vi "SPCC assignment Client.vi"() -> ()   [LabVIEW 2020]
uses:
  Control03.ctl
  Control01.ctl
  Control02.ctl
  <vilib>/regexp/Match Regular Expression.xnode
panel:
  out "error out 5":errorcluster
  out "error out 4":errorcluster
  out "error out 3":errorcluster
  out "error out 2":errorcluster
  out "Enter":T1=enum."disable"
  out "Account number":string
  out "error out":errorcluster
  out "Right Menu 2":string
  out "ATM":string
  out "Right Menu 3":string
  out "Right Menu 1":string
  out "Left Menu 3":string
  out "Left Menu 2":string
  out "Left Menu 1":string
  in  "Right Button 2":bool
  in  "Right Button 3":bool
  in  "Right Button 1":bool
  in  "Left Button 2":bool
  in  "Left Button 3":bool
  in  "Left Button 1":bool
  in  "Enter":bool
  in  "User Input":string
  in  "Card Simulator":bool
  # "ATM Messages"
  # "Right Menu"
  # "Right Buttons"
  # "Left Buttons"
  # "Left Menu"
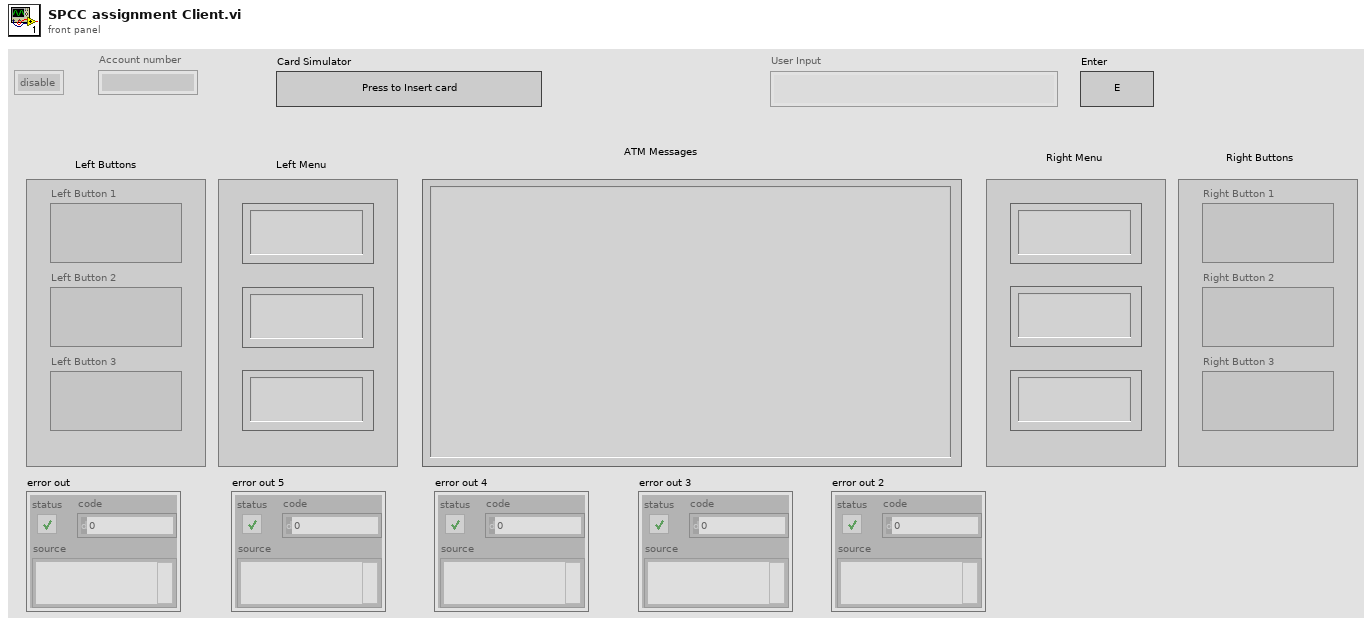
[diagram p1: front panel]
types:
  T1 = typedef "Control03.ctl" = enum16{"withdraw", "deposit", "disable"}
  T2 = typedef "Control01.ctl" = enum16{"Sign in machine", "Start machine", "Welcome "}
  T3 = enum8{"Enabled", "Disabled", "Disabled and Grayed Out"}
  T4 = typedef "Control02.ctl" = enum16{"Start machine", "Welcome "}
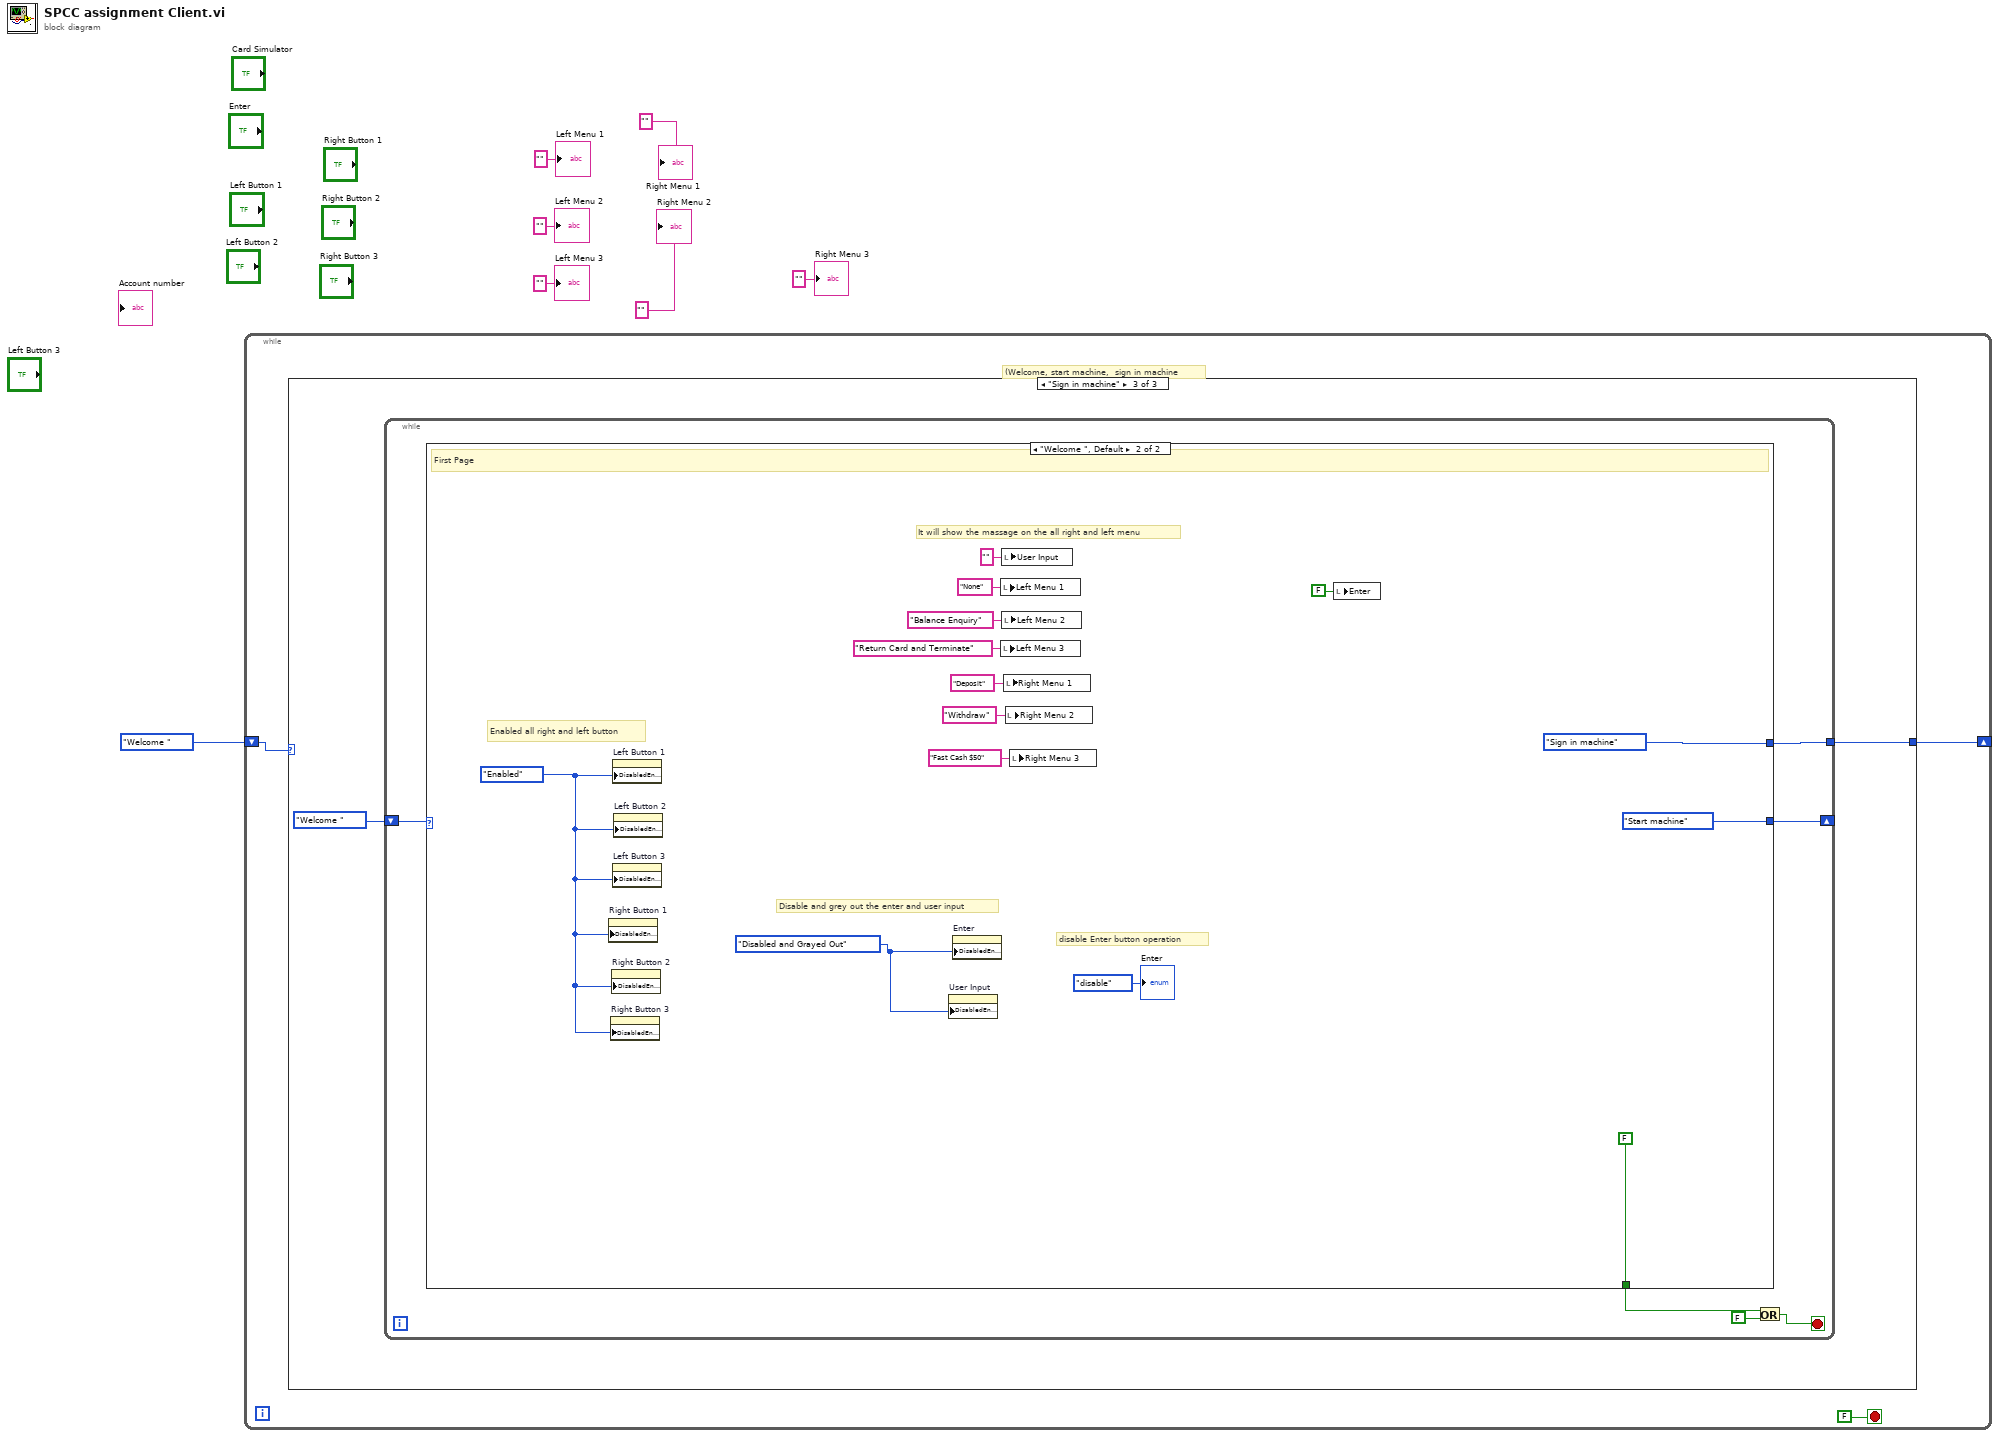
[diagram p0: block diagram]
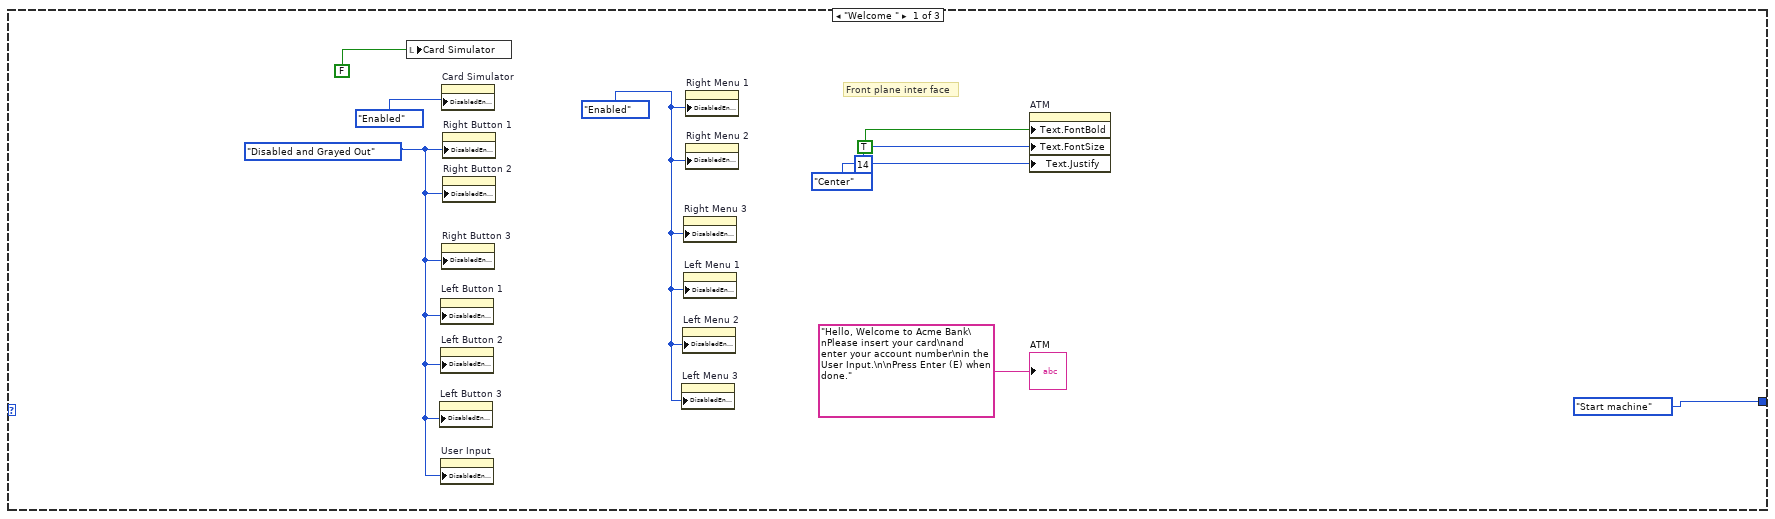
[diagram p2: hidden frame]
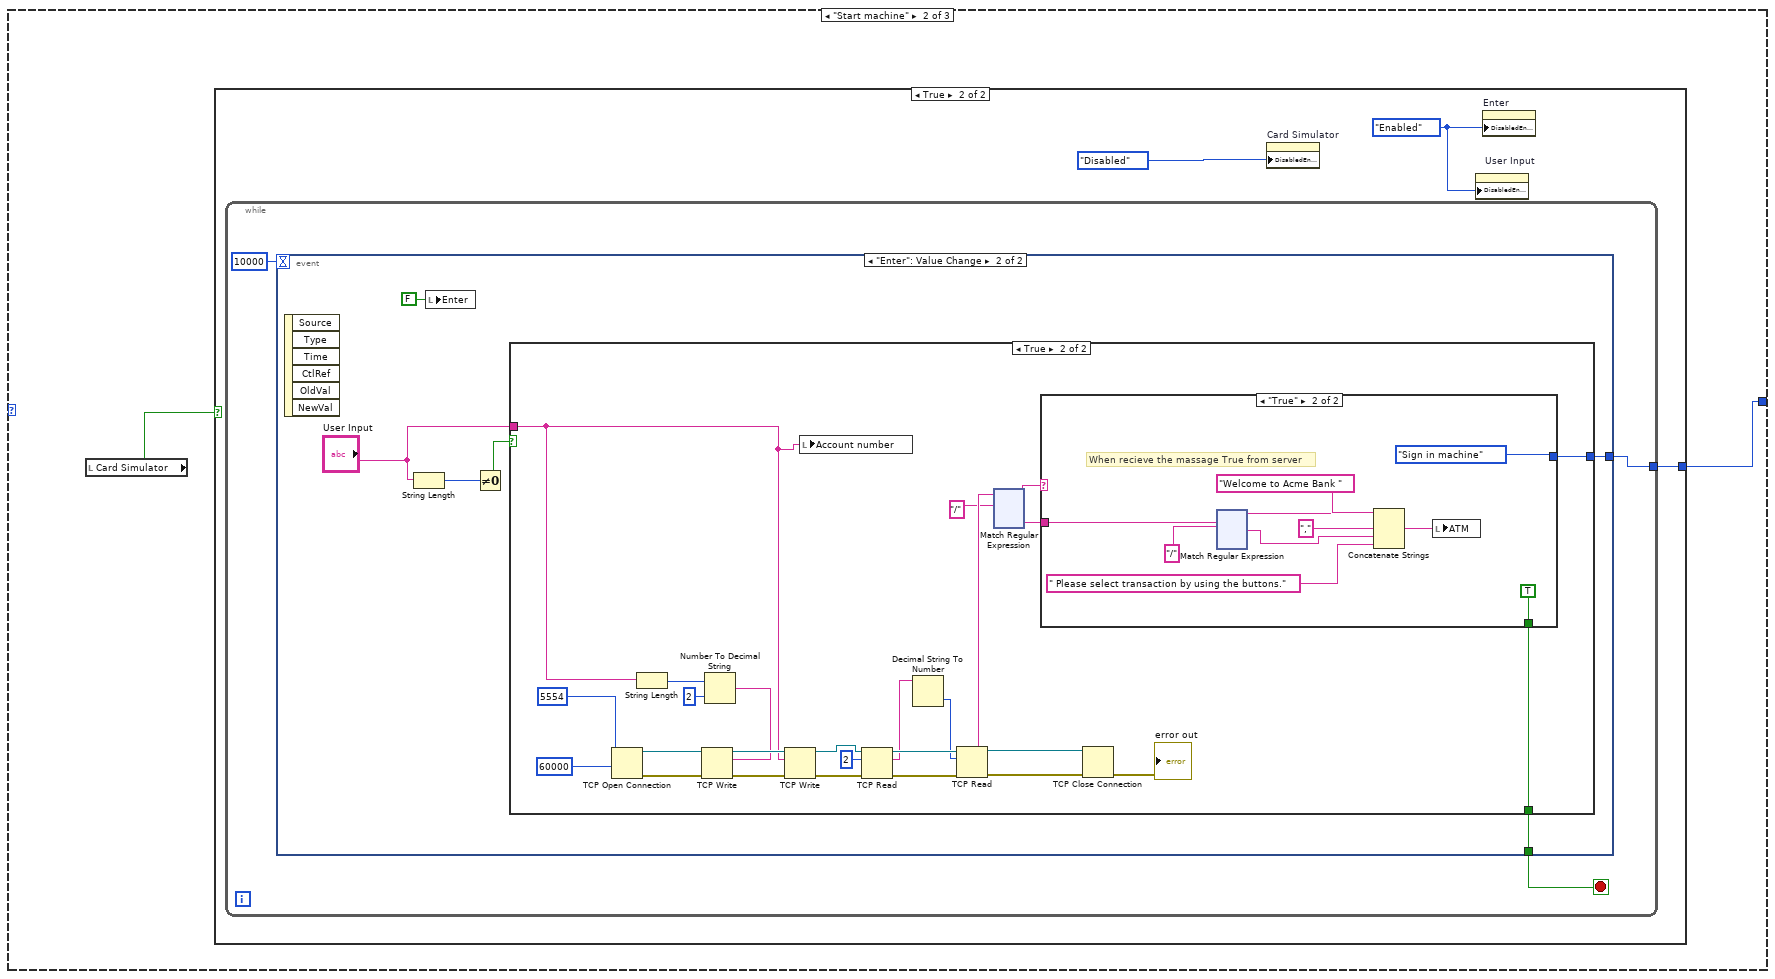
[diagram p3: hidden frame]
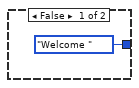
[diagram p4: hidden frame]
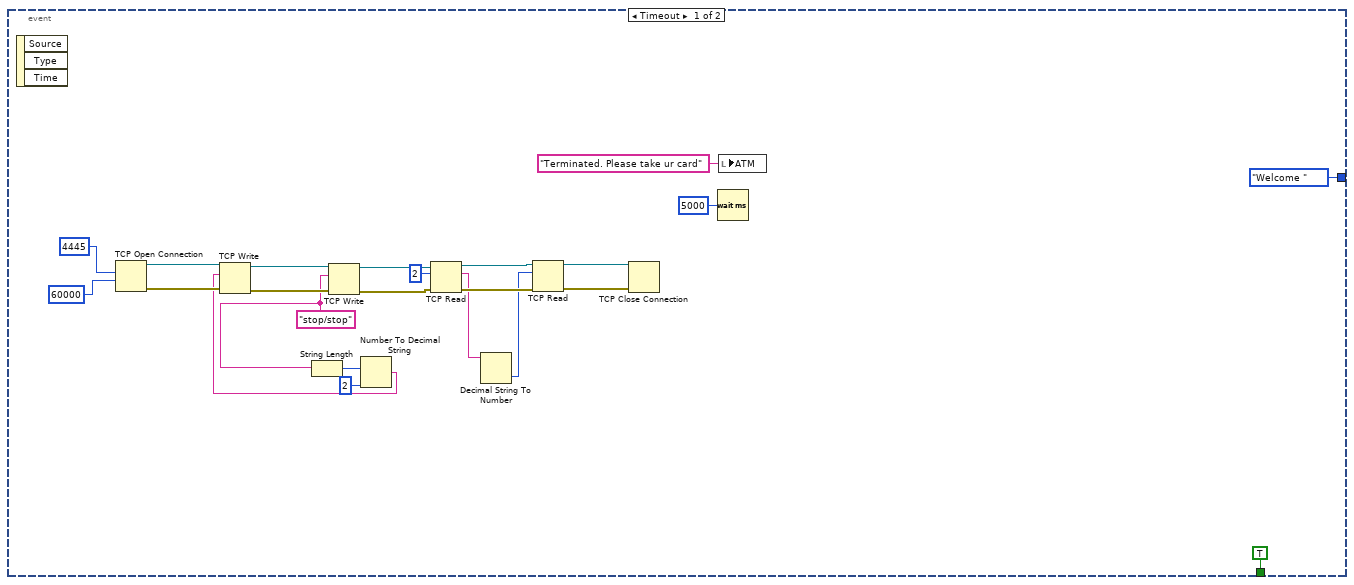
[diagram p5: hidden frame]
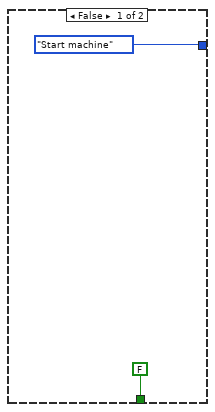
[diagram p6: hidden frame]
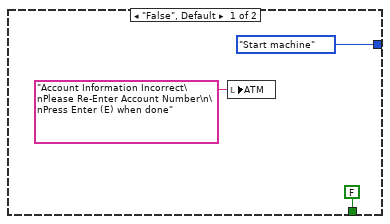
[diagram p7: hidden frame]
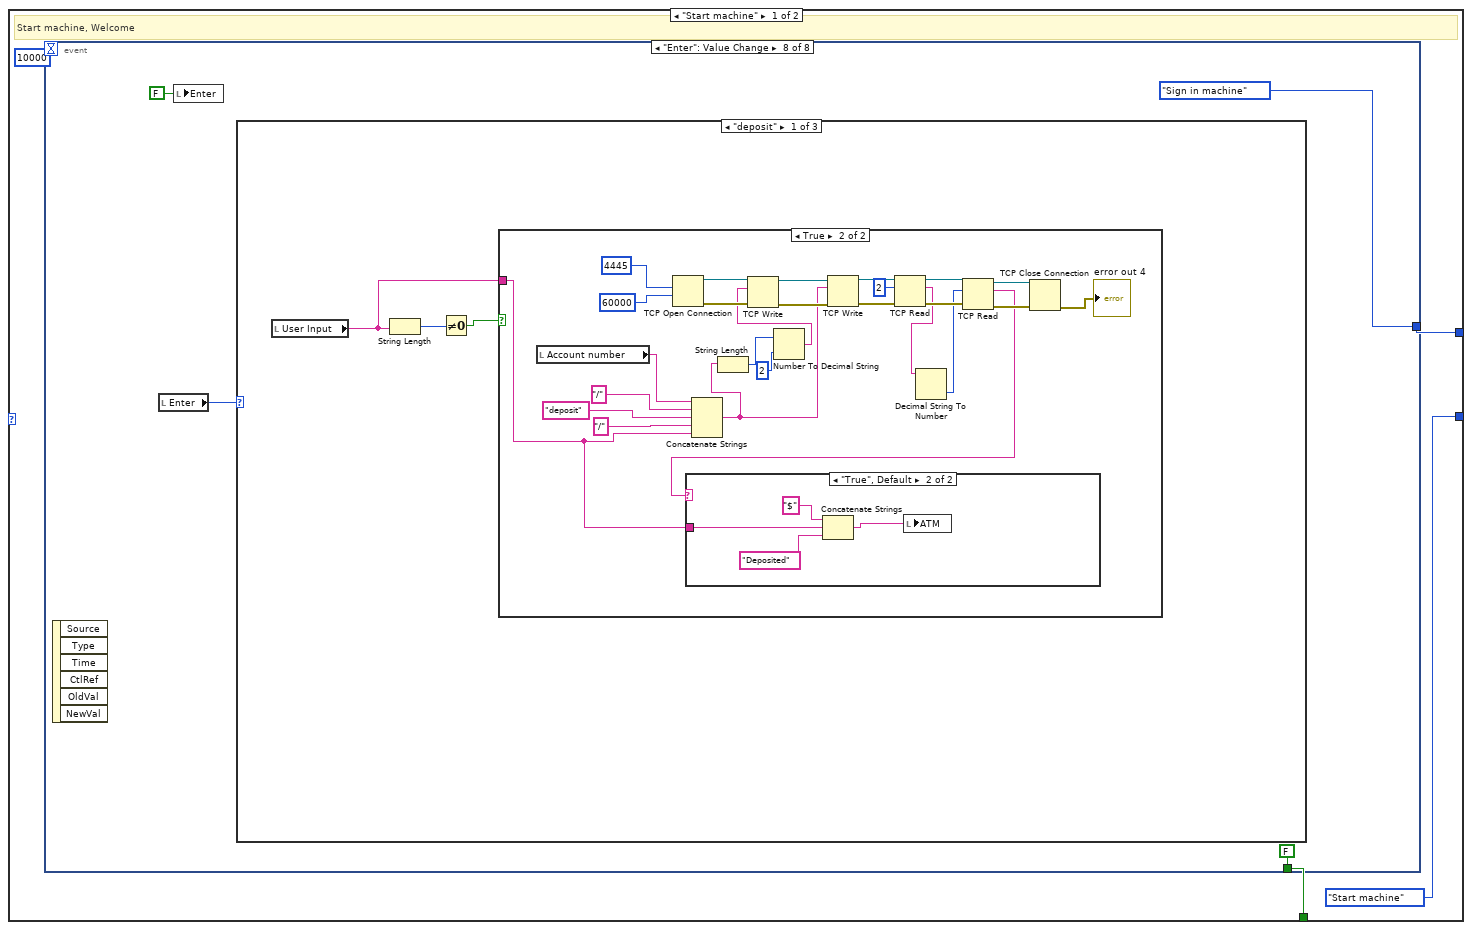
[diagram p8: hidden frame]
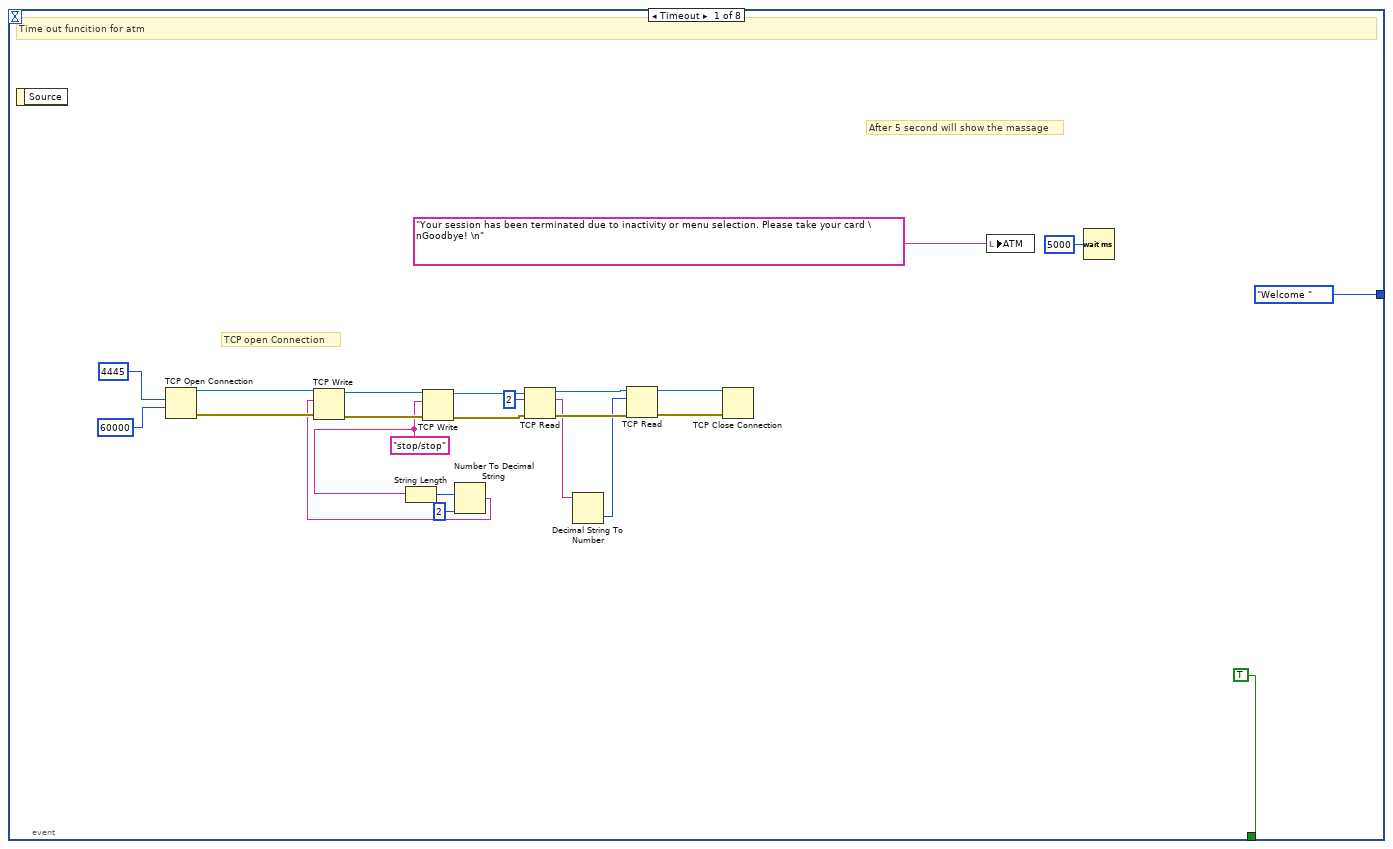
[diagram p9: hidden frame]
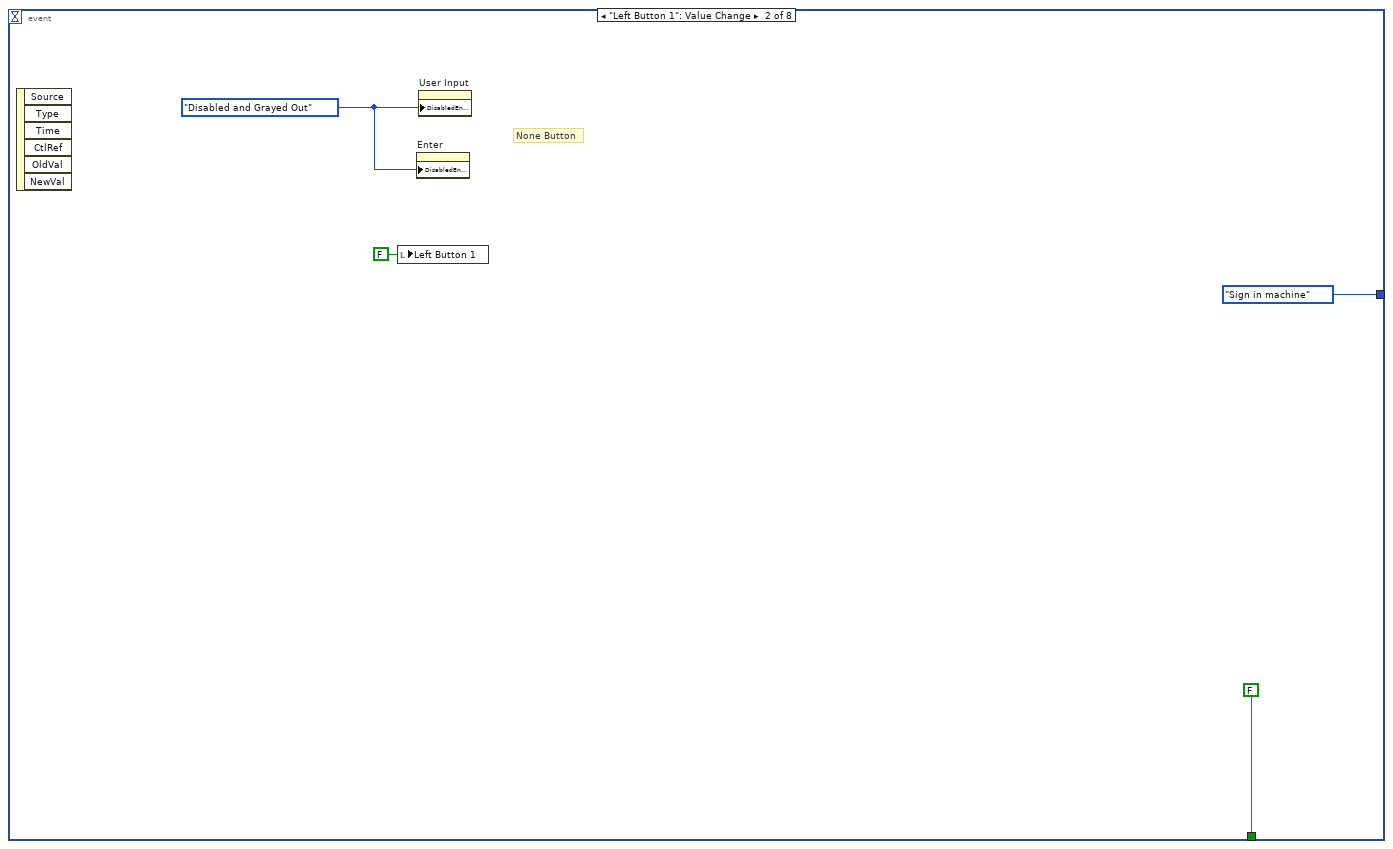
[diagram p10: hidden frame]
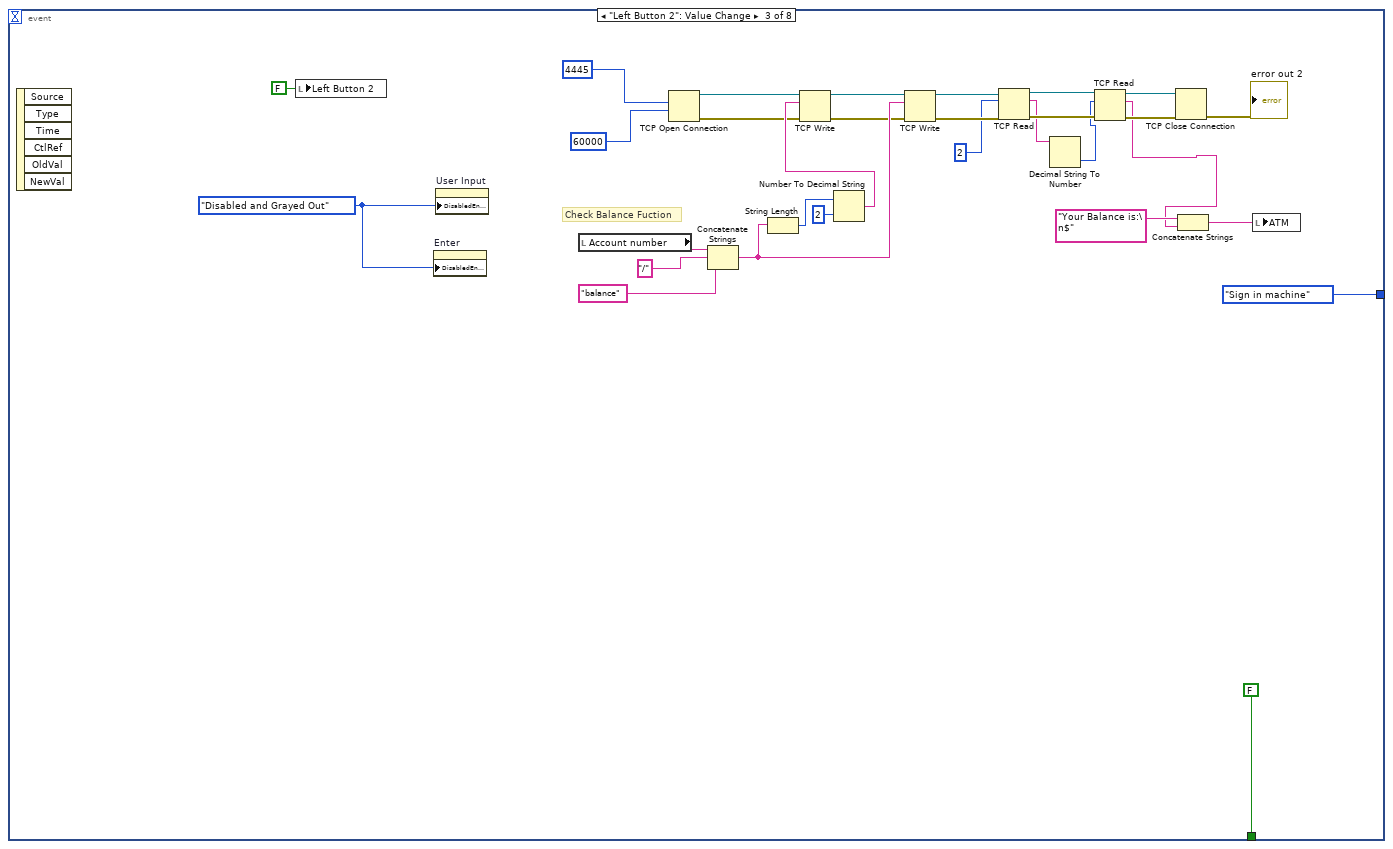
[diagram p11: hidden frame]
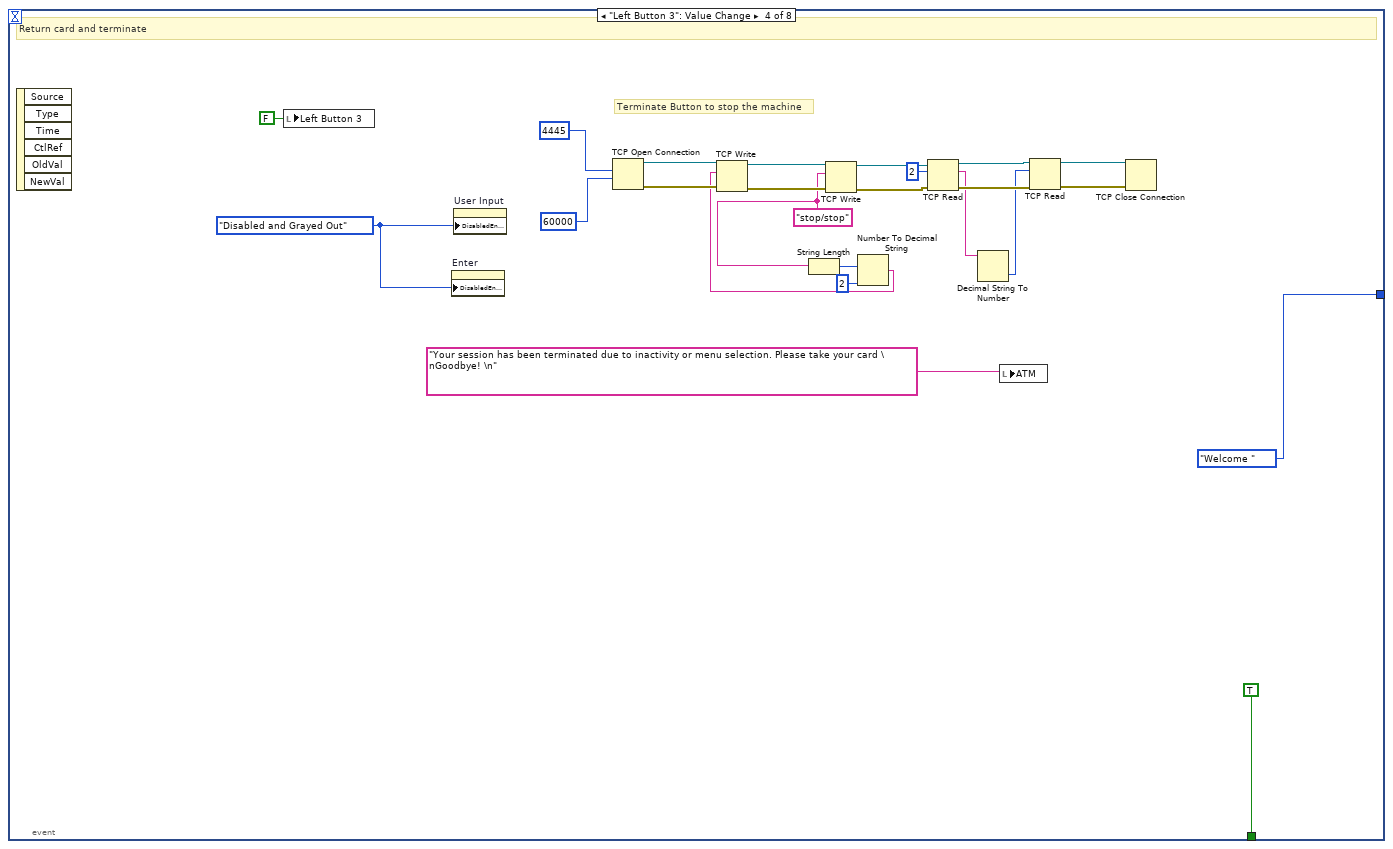
[diagram p12: hidden frame]
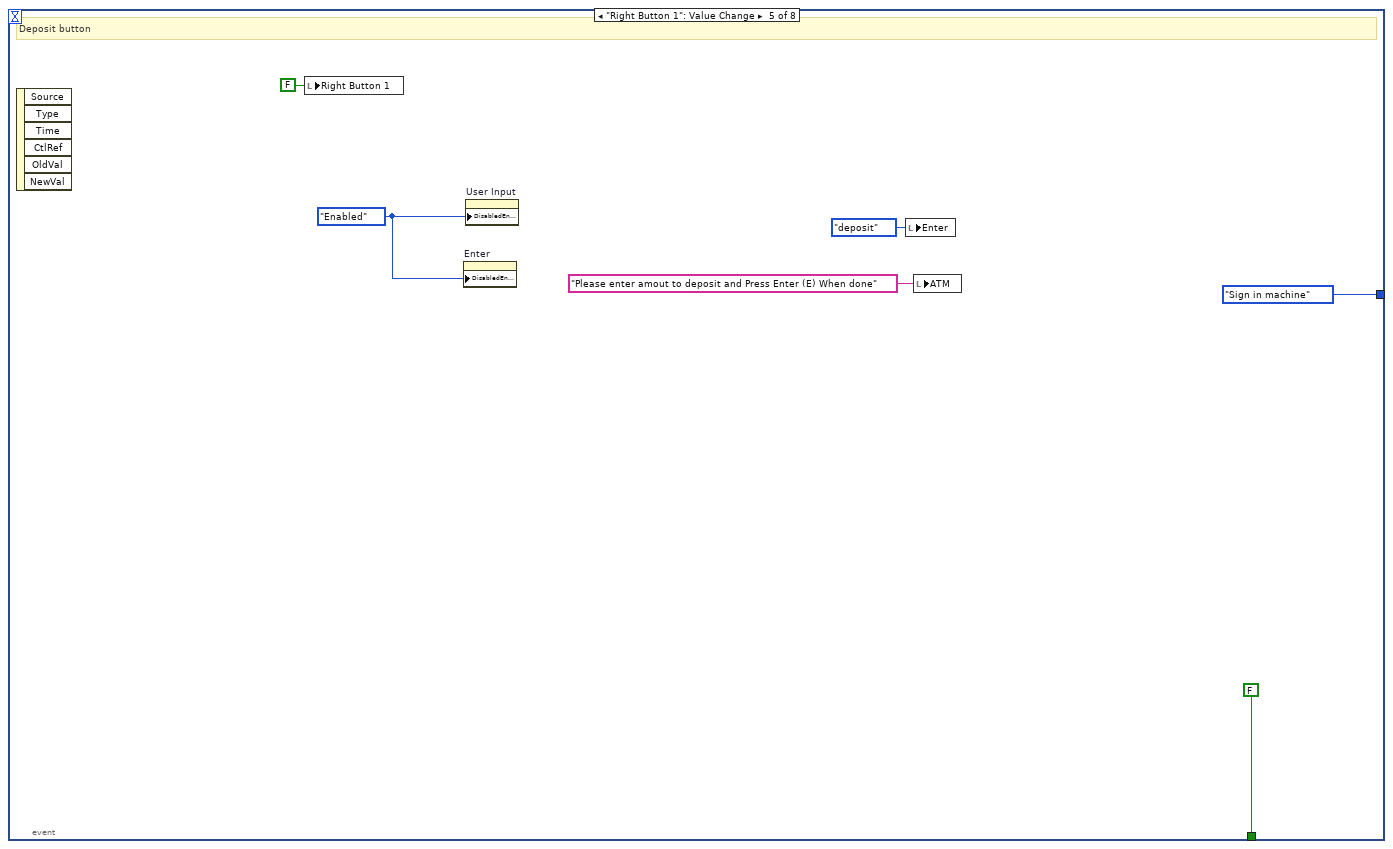
[diagram p13: hidden frame]
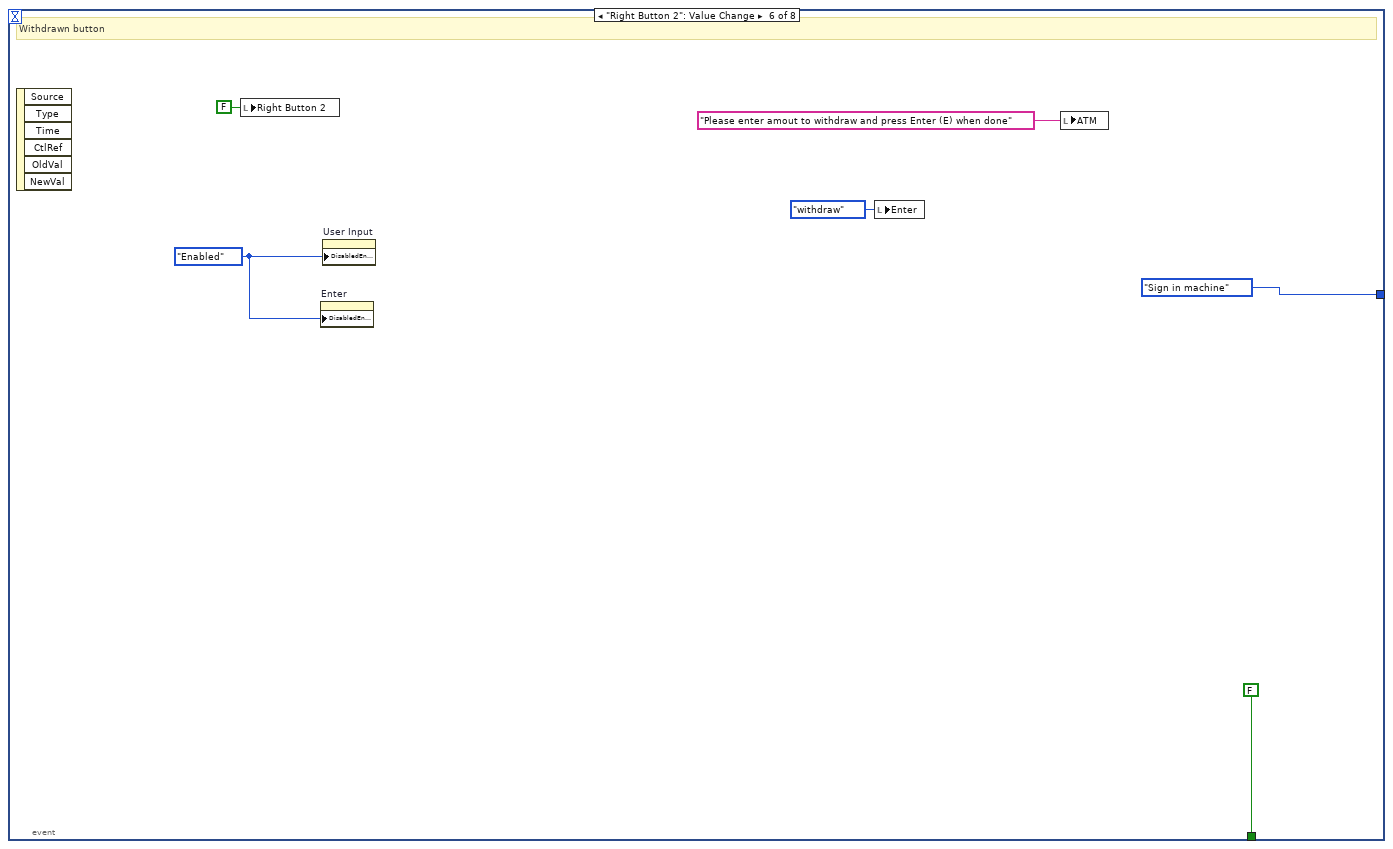
[diagram p14: hidden frame]
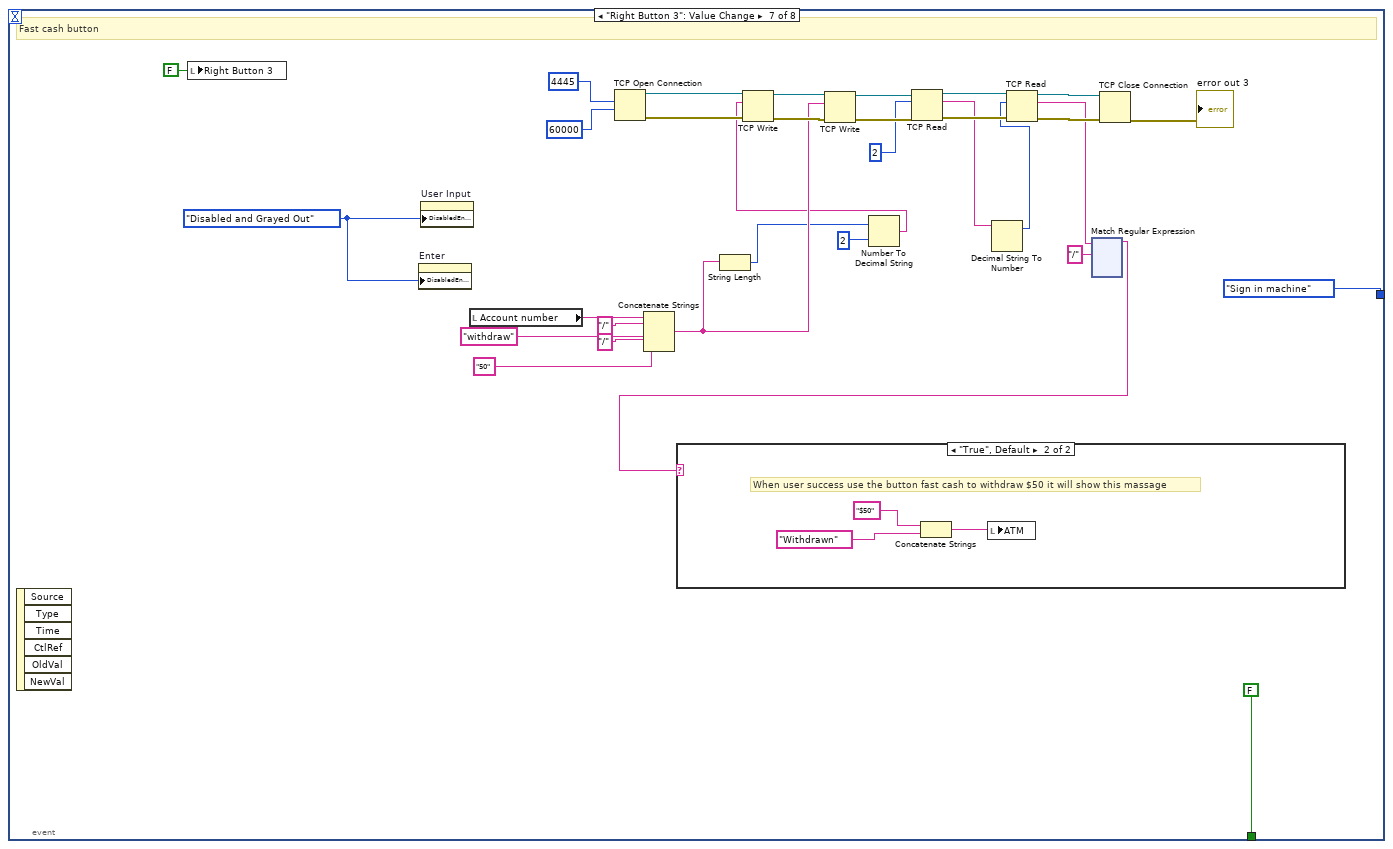
[diagram p15: hidden frame]
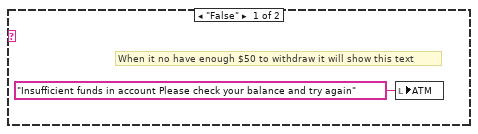
[diagram p16: hidden frame]
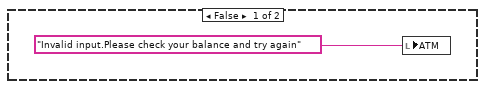
[diagram p17: hidden frame]
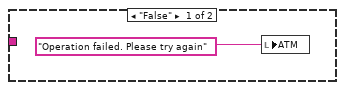
[diagram p18: hidden frame]
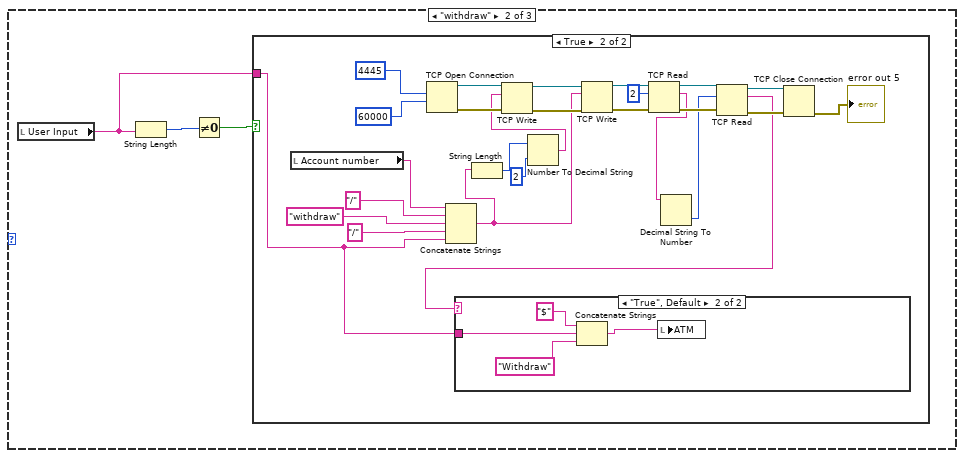
[diagram p19: hidden frame]
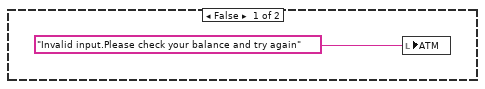
[diagram p20: hidden frame]
diagram:
  n1 = while {
    shift-right: [w8] -> _
    shift-left: Control01."Welcome " ("Enum") -> [w9]
    stop <- FALSE stop-if-true
    # "(Welcome, start machine,  sign in machine"
    n2 = case shown="\"Sign in machine\"" w9 {
      tunnel: [Control01."Start machine" ("Enum") w20 w327] -> w8
      frame "Welcome " {
        w17 = T3."Enabled" ("Disabled")
        w18 = T3."Disabled and Grayed Out" ("Disabled")
        # "Front plane inter face"
        n3 = local write "Card Simulator"(FALSE ("Card Simulator")) -> ()
        n4 = property on="Left Button 3" class="Bool (strict)"("DisabledEnum"=w18) -> ()  [unwired: 2 in, 2 out]
        n5 = property on="Left Button 1" class="Bool (strict)"("DisabledEnum"=w18) -> ()  [unwired: 2 in, 2 out]
        n6 = property on="Left Button 2" class="Bool (strict)"("DisabledEnum"=w18) -> ()  [unwired: 2 in, 2 out]
        n7 = property on="User Input" class="Str"("DisabledEnum"=w18) -> ()  [unwired: 2 in, 2 out]
        n8 = property on="Card Simulator" class="Bool (strict)"("DisabledEnum"=T3."Enabled" ("Disabled")) -> ()  [unwired: 2 in, 2 out]
        n9 = property on="Right Button 3" class="Bool (strict)"("DisabledEnum"=w18) -> ()  [unwired: 2 in, 2 out]
        n10 = property on="Right Button 1" class="Bool (strict)"("DisabledEnum"=w18) -> ()  [unwired: 2 in, 2 out]
        n11 = property on="Right Button 2" class="Bool (strict)"("DisabledEnum"=w18) -> ()  [unwired: 2 in, 2 out]
        n12 = property on="Left Menu 3" class="Str"("DisabledEnum"=w17) -> ()  [unwired: 2 in, 2 out]
        n13 = property on="Left Menu 2" class="Str"("DisabledEnum"=w17) -> ()  [unwired: 2 in, 2 out]
        n14 = property on="Right Menu 3" class="Str"("DisabledEnum"=w17) -> ()  [unwired: 2 in, 2 out]
        n15 = property on="Left Menu 1" class="Str"("DisabledEnum"=w17) -> ()  [unwired: 2 in, 2 out]
        n16 = property on="Right Menu 1" class="Str"("DisabledEnum"=w17) -> ()  [unwired: 2 in, 2 out]
        n17 = property on="Right Menu 2" class="Str"("DisabledEnum"=w17) -> ()  [unwired: 2 in, 2 out]
        n18 = property on="ATM" class="Str"("Text.FontBold"=TRUE ("Text.Font:Bold"), "Text.FontSize"=u32 14 ("Text.Font:Size"), "Text.Justify"=enum16{"Left", "Center", "Right"}."Center" ("Text.Justification")) -> ()  [unwired: 2 in, 2 out]
        "ATM" <- "Hello, Welcome to Acme Bank\nPlease insert your card\nand enter your account number\nin the User Input.\n\nPress Enter (E) when done." ("ATM")
      }
      frame "Start machine" {
        n19 = local read "Card Simulator"() -> (w21:bool)
        n20 = case shown="True" w21 {
          tunnel: [Control01."Welcome " ("Enum") w23] -> w20
          frame False {
          }
          frame True {
            w25 = T3."Enabled" ("Disabled")
            n21 = while {
              tunnel: [w28] -> w23
              stop <- w27 stop-if-true
              n22 = event shown="[1] \"Enter\": Value Change" {
                selector: _ -> [_ _]
                dyn-events: _ -> [_ _]
                timeout: 10000 -> [_ _]
                tunnel: [Control01."Welcome " ("Enum") w54] -> w28
                tunnel: [TRUE w53] -> w27
                event Timeout {
                  w36 = "stop/stop" ("data in")
                  n23 = event-data() -> ()  [unwired: 1 in, 3 out]
                  n24 = TCP Open Connection(remote port or service name=u16 4445, timeout ms (60000)=60000) -> (connection ID=w37:refnum<k5>, error out=w47:errorcluster)  [unwired: 3 in]
                  n25 = String Length(string=w36) -> (length=w31:i32)
                  n26 = Number To Decimal String(number=w31, width (-)=i16 2) -> (decimal integer string=w35:string)
                  n27 = TCP Write(connection ID=w37, data in=w35, error in (no error)=w47) -> (connection ID out=w42:refnum<k5>, error out=w46:errorcluster)  [unwired: 1 in, 1 out]
                  n28 = TCP Write(connection ID=w42, data in=w36, error in (no error)=w46) -> (connection ID out=w41:refnum<k5>, error out=w45:errorcluster)  [unwired: 1 in, 1 out]
                  n29 = TCP Read(connection ID=w41, bytes to read=2, error in (no error)=w45) -> (connection ID out=w40:refnum<k5>, data out=w33:string, error out=w44:errorcluster)  [unwired: 2 in]
                  n30 = Decimal String To Number(string=w33) -> (number=w32:i32)  [unwired: 2 in, 1 out]
                  n31 = TCP Read(connection ID=w40, bytes to read=w32, error in (no error)=w44) -> (connection ID out=w39:refnum<k5>, error out=w43:errorcluster)  [unwired: 2 in, 1 out]
                  n32 = TCP Close Connection(connection ID=w39, error in (no error)=w43) -> ()  [unwired: 1 in, 2 out]
                  n33 = Wait (ms)(milliseconds to wait=u32 5000) -> ()  [unwired: 1 out]
                  n34 = local write "ATM"("Terminated. Please take ur card" ("ATM")) -> ()
                }
                event "Enter": Value Change {
                  n35 = event-data() -> ()  [unwired: 1 in, 6 out]
                  n36 = String Length(string="User Input") -> (length=w57:i32)
                  n37 = local write "Enter"(FALSE ("Enter")) -> ()
                  n38 = Not Equal To 0?(x=w57) -> (x != 0?=w56:bool)
                  n39 = case shown="True" w56 {
                    tunnel: "User Input" -> [_ w66]
                    tunnel: [Control01."Start machine" ("Enum") w61] -> w54
                    tunnel: [FALSE w60] -> w53
                    frame False {
                    }
                    frame True {
                      n40 = TCP Open Connection(remote port or service name=u16 5554, timeout ms (60000)=60000) -> (connection ID=w76:refnum<k5>, error out=w82:errorcluster)  [unwired: 3 in]
                      n41 = String Length(string=w66) -> (length=w85:i32)
                      n42 = Number To Decimal String(number=w85, width (-)=i16 2) -> (decimal integer string=w69:string)
                      n43 = TCP Write(connection ID=w76, data in=w69, error in (no error)=w82) -> (connection ID out=w75:refnum<k5>, error out=w81:errorcluster)  [unwired: 1 in, 1 out]
                      n44 = TCP Write(connection ID=w75, data in=w66, error in (no error)=w81) -> (connection ID out=w74:refnum<k5>, error out=w80:errorcluster)  [unwired: 1 in, 1 out]
                      n45 = local write "Account number"(w66) -> ()
                      n46 = TCP Read(connection ID=w74, bytes to read=2, error in (no error)=w80) -> (connection ID out=w73:refnum<k5>, data out=w71:string, error out=w79:errorcluster)  [unwired: 2 in]
                      n47 = Decimal String To Number(string=w71) -> (number=w70:i32)  [unwired: 2 in, 1 out]
                      n48 = TCP Read(connection ID=w73, bytes to read=w70, error in (no error)=w79) -> (connection ID out=w72:refnum<k5>, data out=w65:string, error out=w78:errorcluster)  [unwired: 2 in]
                      n49 = xnode "Match Regular Expression"("input string"=w65, "regular expression"="/") -> ("before match"=w62:string, "after match"=w63:string)  [unwired: 4 in, 3 out]
                      n50 = case shown="\"True\"" w62 {
                        tunnel: w63 -> [_ w98]
                        tunnel: [FALSE TRUE] -> w60
                        tunnel: [Control01."Start machine" ("Enum") Control01."Sign in machine" ("Enum")] -> w61
                        frame "False", Default {
                          n51 = local write "ATM"("Account Information Incorrect\nPlease Re-Enter Account Number\n\nPress Enter (E) when done" ("ATM")) -> ()
                        }
                        frame "True" {
                          # "When recieve the massage True from server"
                          n52 = xnode "Match Regular Expression"("input string"=w98, "regular expression"="/") -> ("before match"=w95:string, "after match"=w93:string)  [unwired: 4 in, 3 out]
                          n53 = Concatenate Strings("Welcome to Acme Bank " ("string"), w95, "," ("string"), w93, " Please select transaction by using the buttons." ("string")) -> (w91:string)
                          n54 = local write "ATM"(w91) -> ()
                        }
                      }
                      n55 = TCP Close Connection(connection ID=w72, error in (no error)=w78) -> (error out=→"error out":errorcluster)  [unwired: 1 in, 1 out]
                    }
                  }
                }
              }
            }
            n56 = property on="Card Simulator" class="Bool (strict)"("DisabledEnum"=T3."Disabled" ("Disabled")) -> ()  [unwired: 2 in, 2 out]
            n57 = property on="User Input" class="Str"("DisabledEnum"=w25) -> ()  [unwired: 2 in, 2 out]
            n58 = property on="Enter" class="Bool (strict)"("DisabledEnum"=w25) -> ()  [unwired: 2 in, 2 out]
          }
        }
      }
      frame "Sign in machine" {
        # "Welcome, start machine, Sign in machine"
        n59 = while {
          shift-right: [w330] -> _
          shift-left: Control02."Welcome " ("Enum") -> [w331]
          tunnel: [w329] -> w327
          stop <- w334 stop-if-true
          n60 = case shown="\"Welcome \", Default" w331 {
            tunnel: [w338 FALSE ("x")] -> w332
            tunnel: [Control02."Start machine" ("Enum") Control02."Start machine" ("Enum")] -> w330
            tunnel: [w336 Control01."Sign in machine" ("Enum")] -> w329
            frame "Start machine" {
              # "Start machine, Welcome"
              n61 = event shown="[7] \"Enter\": Value Change" {
                selector: _ -> [_ _ _ _ _ _ _ _]
                dyn-events: _ -> [_ _ _ _ _ _ _ _]
                timeout: 10000 -> [_ _ _ _ _ _ _ _]
                tunnel: [TRUE ("x") FALSE ("x") FALSE ("x") TRUE ("x") FALSE ("x") FALSE ("x") FALSE ("x") FALSE ("x")] -> w338
                tunnel: [Control01."Welcome " ("Enum") Control01."Sign in machine" ("Enum") Control01."Sign in machine" ("Enum") Control01."Welcome " ("Enum") Control01."Sign in machine" ("Enum") Control01."Sign in machine" ("Enum") Control01."Sign in machine" ("Enum") Control01."Sign in machine" ("Enum")] -> w336
                event Timeout {
                  w346 = "stop/stop" ("data in")
                  # "TCP open Connection"
                  # "After 5 second will show the massage"
                  # "Time out funcition for atm"
                  n62 = event-data() -> ()  [unwired: 1 in, 1 out]
                  n63 = TCP Open Connection(remote port or service name=u16 4445, timeout ms (60000)=60000) -> (connection ID=w347:refnum<k5>, error out=w357:errorcluster)  [unwired: 3 in]
                  n64 = String Length(string=w346) -> (length=w341:i32)
                  n65 = Number To Decimal String(number=w341, width (-)=i16 2) -> (decimal integer string=w345:string)
                  n66 = TCP Write(connection ID=w347, data in=w345, error in (no error)=w357) -> (connection ID out=w352:refnum<k5>, error out=w356:errorcluster)  [unwired: 1 in, 1 out]
                  n67 = TCP Write(connection ID=w352, data in=w346, error in (no error)=w356) -> (connection ID out=w351:refnum<k5>, error out=w355:errorcluster)  [unwired: 1 in, 1 out]
                  n68 = TCP Read(connection ID=w351, bytes to read=2, error in (no error)=w355) -> (connection ID out=w350:refnum<k5>, data out=w343:string, error out=w354:errorcluster)  [unwired: 2 in]
                  n69 = Decimal String To Number(string=w343) -> (number=w342:i32)  [unwired: 2 in, 1 out]
                  n70 = TCP Read(connection ID=w350, bytes to read=w342, error in (no error)=w354) -> (connection ID out=w349:refnum<k5>, error out=w353:errorcluster)  [unwired: 2 in, 1 out]
                  n71 = TCP Close Connection(connection ID=w349, error in (no error)=w353) -> ()  [unwired: 1 in, 2 out]
                  n72 = local write "ATM"("Your session has been terminated due to inactivity or menu selection. Please take your card \nGoodbye! \n" ("ATM")) -> ()
                  n73 = Wait (ms)(milliseconds to wait=u32 5000) -> ()  [unwired: 1 out]
                }
                event "Left Button 1": Value Change {
                  w364 = T3."Disabled and Grayed Out" ("Disabled")
                  # "None Button"
                  n74 = event-data() -> ()  [unwired: 1 in, 6 out]
                  n75 = local write "Left Button 1"(FALSE ("Left Button 1")) -> ()
                  n76 = property on="Enter" class="Bool (strict)"("DisabledEnum"=w364) -> ()  [unwired: 2 in, 2 out]
                  n77 = property on="User Input" class="Str"("DisabledEnum"=w364) -> ()  [unwired: 2 in, 2 out]
                }
                event "Left Button 2": Value Change {
                  w394 = T3."Disabled and Grayed Out" ("Disabled")
                  # "Check Balance Fuction"
                  n78 = event-data() -> ()  [unwired: 1 in, 6 out]
                  n79 = local write "Left Button 2"(FALSE ("Left Button 2")) -> ()
                  n80 = property on="Enter" class="Bool (strict)"("DisabledEnum"=w394) -> ()  [unwired: 2 in, 2 out]
                  n81 = property on="User Input" class="Str"("DisabledEnum"=w394) -> ()  [unwired: 2 in, 2 out]
                  n82 = local read "Account number"() -> (w392:string)
                  n83 = TCP Open Connection(remote port or service name=u16 4445, timeout ms (60000)=60000) -> (connection ID=w384:refnum<k5>, error out=w379:errorcluster)  [unwired: 3 in]
                  n84 = Concatenate Strings(w392, "/" ("string"), "balance" ("string")) -> (w389:string)
                  n85 = String Length(string=w389) -> (length=w388:i32)
                  n86 = Number To Decimal String(number=w388, width (-)=i16 2) -> (decimal integer string=w386:string)
                  n87 = TCP Write(connection ID=w384, data in=w386, error in (no error)=w379) -> (connection ID out=w383:refnum<k5>, error out=w378:errorcluster)  [unwired: 1 in, 1 out]
                  n88 = TCP Write(connection ID=w383, data in=w389, error in (no error)=w378) -> (connection ID out=w382:refnum<k5>, error out=w377:errorcluster)  [unwired: 1 in, 1 out]
                  n89 = TCP Read(connection ID=w382, bytes to read=2, error in (no error)=w377) -> (connection ID out=w381:refnum<k5>, data out=w372:string, error out=w376:errorcluster)  [unwired: 2 in]
                  n90 = Decimal String To Number(string=w372) -> (number=w371:i32)  [unwired: 2 in, 1 out]
                  n91 = TCP Read(connection ID=w381, bytes to read=w371, error in (no error)=w376) -> (connection ID out=w380:refnum<k5>, data out=w367:string, error out=w375:errorcluster)  [unwired: 2 in]
                  n92 = TCP Close Connection(connection ID=w380, error in (no error)=w375) -> (error out=→"error out 2":errorcluster)  [unwired: 1 in, 1 out]
                  n93 = Concatenate Strings("Your Balance is:\n$" ("string"), w367) -> (w369:string)
                  n94 = local write "ATM"(w369) -> ()
                }
                event "Left Button 3": Value Change {
                  w405 = "stop/stop" ("data in")
                  w417 = T3."Disabled and Grayed Out" ("Disabled")
                  # "Terminate Button to stop the machine"
                  # "Return card and terminate"
                  n95 = event-data() -> ()  [unwired: 1 in, 6 out]
                  n96 = local write "Left Button 3"(FALSE ("Left Button 3")) -> ()
                  n97 = property on="Enter" class="Bool (strict)"("DisabledEnum"=w417) -> ()  [unwired: 2 in, 2 out]
                  n98 = property on="User Input" class="Str"("DisabledEnum"=w417) -> ()  [unwired: 2 in, 2 out]
                  n99 = TCP Open Connection(remote port or service name=u16 4445, timeout ms (60000)=60000) -> (connection ID=w406:refnum<k5>, error out=w416:errorcluster)  [unwired: 3 in]
                  n100 = String Length(string=w405) -> (length=w400:i32)
                  n101 = Number To Decimal String(number=w400, width (-)=i16 2) -> (decimal integer string=w404:string)
                  n102 = TCP Write(connection ID=w406, data in=w404, error in (no error)=w416) -> (connection ID out=w411:refnum<k5>, error out=w415:errorcluster)  [unwired: 1 in, 1 out]
                  n103 = TCP Write(connection ID=w411, data in=w405, error in (no error)=w415) -> (connection ID out=w410:refnum<k5>, error out=w414:errorcluster)  [unwired: 1 in, 1 out]
                  n104 = TCP Read(connection ID=w410, bytes to read=2, error in (no error)=w414) -> (connection ID out=w409:refnum<k5>, data out=w402:string, error out=w413:errorcluster)  [unwired: 2 in]
                  n105 = Decimal String To Number(string=w402) -> (number=w401:i32)  [unwired: 2 in, 1 out]
                  n106 = local write "ATM"("Your session has been terminated due to inactivity or menu selection. Please take your card \nGoodbye! \n" ("ATM")) -> ()
                  n107 = TCP Read(connection ID=w409, bytes to read=w401, error in (no error)=w413) -> (connection ID out=w408:refnum<k5>, error out=w412:errorcluster)  [unwired: 2 in, 1 out]
                  n108 = TCP Close Connection(connection ID=w408, error in (no error)=w412) -> ()  [unwired: 1 in, 2 out]
                }
                event "Right Button 1": Value Change {
                  w422 = T3."Enabled" ("Disabled")
                  # "Deposit button"
                  n109 = event-data() -> ()  [unwired: 1 in, 6 out]
                  n110 = local write "Right Button 1"(FALSE ("Right Button 1")) -> ()
                  n111 = property on="Enter" class="Bool (strict)"("DisabledEnum"=w422) -> ()  [unwired: 2 in, 2 out]
                  n112 = property on="User Input" class="Str"("DisabledEnum"=w422) -> ()  [unwired: 2 in, 2 out]
                  n113 = local write "Enter"(Control03."deposit" ("Enter")) -> ()
                  n114 = local write "ATM"("Please enter amout to deposit and Press Enter (E) When done" ("ATM")) -> ()
                }
                event "Right Button 2": Value Change {
                  w428 = T3."Enabled" ("Disabled")
                  # "Withdrawn button"
                  n115 = event-data() -> ()  [unwired: 1 in, 6 out]
                  n116 = local write "Right Button 2"(FALSE ("Right Button 2")) -> ()
                  n117 = property on="Enter" class="Bool (strict)"("DisabledEnum"=w428) -> ()  [unwired: 2 in, 2 out]
                  n118 = property on="User Input" class="Str"("DisabledEnum"=w428) -> ()  [unwired: 2 in, 2 out]
                  n119 = local write "Enter"(Control03."withdraw" ("Enter")) -> ()
                  n120 = local write "ATM"("Please enter amout to withdraw and press Enter (E) when done" ("ATM")) -> ()
                }
                event "Right Button 3": Value Change {
                  w462 = T3."Disabled and Grayed Out" ("Disabled")
                  # "Fast cash button"
                  n121 = event-data() -> ()  [unwired: 1 in, 6 out]
                  n122 = local write "Right Button 3"(FALSE ("Right Button 3")) -> ()
                  n123 = property on="Enter" class="Bool (strict)"("DisabledEnum"=w462) -> ()  [unwired: 2 in, 2 out]
                  n124 = property on="User Input" class="Str"("DisabledEnum"=w462) -> ()  [unwired: 2 in, 2 out]
                  n125 = local read "Account number"() -> (w449:string)
                  n126 = TCP Open Connection(remote port or service name=u16 4445, timeout ms (60000)=60000) -> (connection ID=w460:refnum<k5>, error out=w456:errorcluster)  [unwired: 3 in]
                  n127 = Concatenate Strings(w449, "/" ("string"), "withdraw" ("string"), "/" ("string"), "50" ("string")) -> (w444:string)
                  n128 = String Length(string=w444) -> (length=w443:i32)
                  n129 = Number To Decimal String(number=w443, width (-)=i16 2) -> (decimal integer string=w441:string)
                  n130 = TCP Write(connection ID=w460, data in=w441, error in (no error)=w456) -> (connection ID out=w459:refnum<k5>, error out=w455:errorcluster)  [unwired: 1 in, 1 out]
                  n131 = TCP Write(connection ID=w459, data in=w444, error in (no error)=w455) -> (connection ID out=w440:refnum<k5>, error out=w454:errorcluster)  [unwired: 1 in, 1 out]
                  n132 = TCP Read(connection ID=w440, bytes to read=2, error in (no error)=w454) -> (connection ID out=w458:refnum<k5>, data out=w438:string, error out=w453:errorcluster)  [unwired: 2 in]
                  n133 = Decimal String To Number(string=w438) -> (offset past number=w437:i32)  [unwired: 2 in, 1 out]
                  n134 = TCP Read(connection ID=w458, bytes to read=w437, error in (no error)=w453) -> (connection ID out=w457:refnum<k5>, data out=w436:string, error out=w452:errorcluster)  [unwired: 2 in]
                  n135 = xnode "Match Regular Expression"("input string"=w436, "regular expression"="/") -> ("before match"=w434:string)  [unwired: 4 in, 4 out]
                  n136 = case shown="\"True\", Default" w434 {
                    frame "False" {
                      # "When it no have enough $50 to withdraw it will show this text"
                      n137 = local write "ATM"("Insufficient funds in account Please check your balance and try again" ("ATM")) -> ()
                    }
                    frame "True", Default {
                      # "When user success use the button fast cash to withdraw $50 it will show this massage"
                      n138 = Concatenate Strings("$50" ("string"), "Withdrawn" ("string")) -> (w465:string)
                      n139 = local write "ATM"(w465) -> ()
                    }
                  }
                  n140 = TCP Close Connection(connection ID=w457, error in (no error)=w452) -> (error out=→"error out 3":errorcluster)  [unwired: 1 in, 1 out]
                }
                event "Enter": Value Change {
                  n141 = event-data() -> ()  [unwired: 1 in, 6 out]
                  n142 = local read "Enter"() -> (w585:T1)
                  n143 = local write "Enter"(FALSE ("Enter")) -> ()
                  n144 = case shown="\"deposit\"" w585 {
                    frame "deposit" {
                      n145 = local read "User Input"() -> (w586:string)
                      n146 = String Length(string=w586) -> (length=w588:i32)
                      n147 = Not Equal To 0?(x=w588) -> (x != 0?=w587:bool)
                      n148 = case shown="True" w587 {
                        tunnel: w586 -> [_ w591]
                        frame False {
                          n149 = local write "ATM"("Invalid input.Please check your balance and try again" ("ATM")) -> ()
                        }
                        frame True {
                          n150 = local read "Account number"() -> (w615:string)
                          n151 = TCP Open Connection(remote port or service name=u16 4445, timeout ms (60000)=60000) -> (connection ID=w605:refnum<k5>, error out=w611:errorcluster)  [unwired: 3 in]
                          n152 = Concatenate Strings(w615, "/" ("string"), "deposit" ("string"), "/" ("string"), w591) -> (w598:string)
                          n153 = String Length(string=w598) -> (length=w600:i32)
                          n154 = Number To Decimal String(number=w600, width (-)=i16 2) -> (decimal integer string=w597:string)
                          n155 = TCP Write(connection ID=w605, data in=w597, error in (no error)=w611) -> (connection ID out=w604:refnum<k5>, error out=w610:errorcluster)  [unwired: 1 in, 1 out]
                          n156 = TCP Write(connection ID=w604, data in=w598, error in (no error)=w610) -> (connection ID out=w603:refnum<k5>, error out=w609:errorcluster)  [unwired: 1 in, 1 out]
                          n157 = TCP Read(connection ID=w603, bytes to read=2, error in (no error)=w609) -> (connection ID out=w602:refnum<k5>, data out=w593:string, error out=w608:errorcluster)  [unwired: 2 in]
                          n158 = Decimal String To Number(string=w593) -> (number=w592:i32)  [unwired: 2 in, 1 out]
                          n159 = TCP Read(connection ID=w602, bytes to read=w592, error in (no error)=w608) -> (connection ID out=w601:refnum<k5>, data out=w595:string, error out=w607:errorcluster)  [unwired: 2 in]
                          n160 = case shown="\"True\", Default" w595 {
                            tunnel: w591 -> [_ w617]
                            frame "False" {
                              n161 = local write "ATM"("Operation failed. Please try again" ("ATM")) -> ()
                            }
                            frame "True", Default {
                              n162 = Concatenate Strings("$" ("string"), w617, "Deposited" ("string")) -> (w618:string)
                              n163 = local write "ATM"(w618) -> ()
                            }
                          }
                          n164 = TCP Close Connection(connection ID=w601, error in (no error)=w607) -> (error out=→"error out 4":errorcluster)  [unwired: 1 in, 1 out]
                        }
                      }
                    }
                    frame "withdraw" {
                      n165 = local read "User Input"() -> (w621:string)
                      n166 = String Length(string=w621) -> (length=w623:i32)
                      n167 = Not Equal To 0?(x=w623) -> (x != 0?=w622:bool)
                      n168 = case shown="True" w622 {
                        tunnel: w621 -> [_ w626]
                        frame False {
                          n169 = local write "ATM"("Invalid input.Please check your balance and try again" ("ATM")) -> ()
                        }
                        frame True {
                          n170 = local read "Account number"() -> (w650:string)
                          n171 = TCP Open Connection(remote port or service name=u16 4445, timeout ms (60000)=60000) -> (connection ID=w640:refnum<k5>, error out=w646:errorcluster)  [unwired: 3 in]
                          n172 = Concatenate Strings(w650, "/" ("string"), "withdraw" ("string"), "/" ("string"), w626) -> (w633:string)
                          n173 = String Length(string=w633) -> (length=w635:i32)
                          n174 = Number To Decimal String(number=w635, width (-)=i16 2) -> (decimal integer string=w632:string)
                          n175 = TCP Write(connection ID=w640, data in=w632, error in (no error)=w646) -> (connection ID out=w639:refnum<k5>, error out=w645:errorcluster)  [unwired: 1 in, 1 out]
                          n176 = TCP Write(connection ID=w639, data in=w633, error in (no error)=w645) -> (connection ID out=w638:refnum<k5>, error out=w644:errorcluster)  [unwired: 1 in, 1 out]
                          n177 = TCP Read(connection ID=w638, bytes to read=2, error in (no error)=w644) -> (connection ID out=w637:refnum<k5>, data out=w627:string, error out=w643:errorcluster)  [unwired: 2 in]
                          n178 = Decimal String To Number(string=w627) -> (number=w630:i32)  [unwired: 2 in, 1 out]
                          n179 = TCP Read(connection ID=w637, bytes to read=w630, error in (no error)=w643) -> (connection ID out=w636:refnum<k5>, data out=w629:string, error out=w642:errorcluster)  [unwired: 2 in]
                          n180 = case shown="\"True\", Default" w629 {
                            tunnel: w626 -> [_ w652]
                            frame "False" {
                              n181 = local write "ATM"("Insufficient funds in account Please check your balance and try again" ("ATM")) -> ()
                            }
                            frame "True", Default {
                              n182 = Concatenate Strings("$" ("string"), w652, "Withdraw" ("string")) -> (w653:string)
                              n183 = local write "ATM"(w653) -> ()
                            }
                          }
                          n184 = TCP Close Connection(connection ID=w636, error in (no error)=w642) -> (error out=→"error out 5":errorcluster)  [unwired: 1 in, 1 out]
                        }
                      }
                    }
                    frame "disable", Default {
                    }
                  }
                }
              }
            }
            frame "Welcome ", Default {
              w659 = T3."Disabled and Grayed Out" ("Disabled")
              w669 = T3."Enabled" ("Disabled")
              # "It will show the massage on the all right and left menu"
              # "disable Enter button operation"
              # "Disable and grey out the enter and user input"
              # "Enabled all right and left button"
              # "First Page"
              n185 = property on="Right Button 1" class="Bool (strict)"("DisabledEnum"=w669) -> ()  [unwired: 2 in, 2 out]
              n186 = property on="Right Button 3" class="Bool (strict)"("DisabledEnum"=w669) -> ()  [unwired: 2 in, 2 out]
              n187 = property on="Right Button 2" class="Bool (strict)"("DisabledEnum"=w669) -> ()  [unwired: 2 in, 2 out]
              n188 = property on="Left Button 1" class="Bool (strict)"("DisabledEnum"=w669) -> ()  [unwired: 2 in, 2 out]
              n189 = property on="Left Button 3" class="Bool (strict)"("DisabledEnum"=w669) -> ()  [unwired: 2 in, 2 out]
              n190 = property on="Left Button 2" class="Bool (strict)"("DisabledEnum"=w669) -> ()  [unwired: 2 in, 2 out]
              n191 = property on="User Input" class="Str"("DisabledEnum"=w659) -> ()  [unwired: 2 in, 2 out]
              n192 = property on="Enter" class="Bool (strict)"("DisabledEnum"=w659) -> ()  [unwired: 2 in, 2 out]
              n193 = local write "Left Menu 1"("None" ("Left Menu 1")) -> ()
              n194 = local write "Left Menu 3"("Return Card and Terminate" ("Left Menu 3")) -> ()
              n195 = local write "User Input"("" ("User Input")) -> ()
              n196 = local write "Left Menu 2"("Balance Enquiry" ("Left Menu 2")) -> ()
              n197 = local write "Right Menu 1"("Deposit" ("Right Menu 1")) -> ()
              n198 = local write "Right Menu 2"("Withdraw" ("Right Menu 2")) -> ()
              n199 = local write "Right Menu 3"("Fast Cash $50" ("Right Menu 3")) -> ()
              n200 = local write "Enter"(FALSE ("Enter")) -> ()
              "Enter" <- Control03."disable"
            }
          }
          n201 = Or(x=w332, y=FALSE) -> (x .or. y?=w334:bool)
        }
      }
    }
  }
  "Left Menu 1" <- "" ("Left Menu 1")
  "Left Menu 2" <- "" ("Left Menu 2")
  "Left Menu 3" <- "" ("Left Menu 3")
  "Right Menu 1" <- "" ("Right Menu 1")
  "Right Menu 3" <- "" ("Right Menu 3")
  "Right Menu 2" <- "" ("Right Menu 2")
